vi "TPSConnect2_Test.vi"() -> ()   [LabVIEW 2009]
panel:
  in  "stop":bool
  out "Array":dbl[](array[numeric])
  in  "error in (no error)":errorcluster
  out "error out":errorcluster
  in  "ip":string
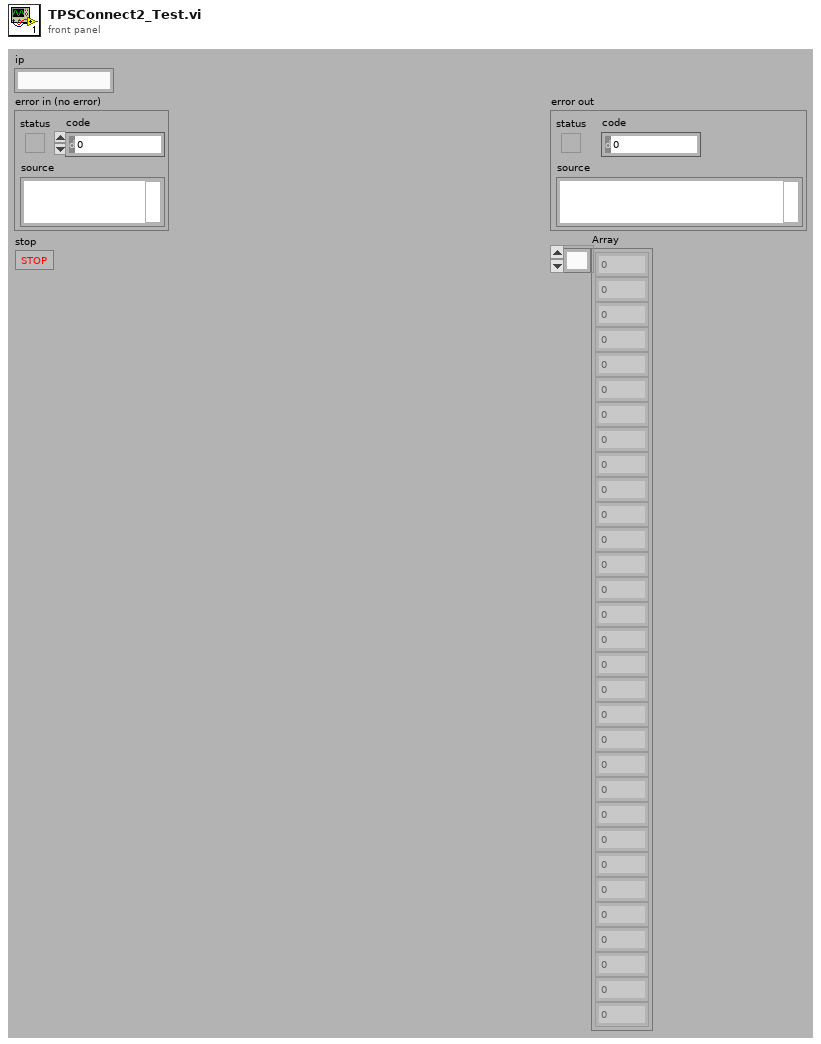
[diagram p1: front panel]
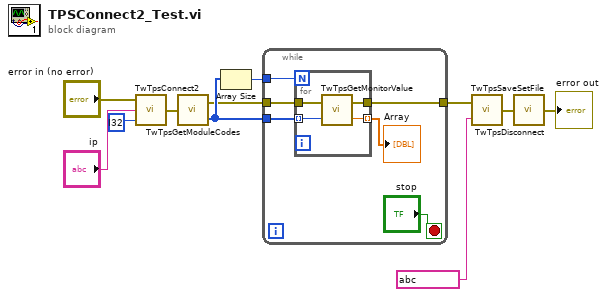
[diagram p0: block diagram]
diagram:
  n1 = call "TwTpsConnect2.vi"("type"=i32 ?, "ip"="ip", "error in (no error)"="error in (no error)") -> ("error out"=w9:errorcluster)
  n2 = call "TwTpsGetModuleCodes.vi"("error in (no error)"=w9) -> ("error out"=w5:errorcluster, "moduleCodeBuffer"=w6:i32[])
  n3 = Array Size(array=w6) -> (size(s)=w7:i32)
  n4 = while {
    tunnel: w7 -> [w17]
    tunnel: w6 -> [w16]
    tunnel: w5 -> [w15]
    tunnel: [w14] -> w3
    stop <- "stop" stop-if-true
    n5 = for {
      N: w17 -> [_]
      tunnel: w16 -> [w19] mode=indexing
      tunnel: w15 -> [w21]
      tunnel: [w20] -> w14
      tunnel: [w18] -> w12 mode=indexing
      n6 = call "TwTpsGetMonitorValue.vi"("moduleCode"=w19, "error in (no error)"=w21) -> ("value"=w18:dbl, "error out"=w20:errorcluster)
    }
    "Array" <- w12
  }
  n7 = call "TwTpsSaveSetFile.vi"("setFile"=string ?, "error in (no error)"=w3) -> ("error out"=w2:errorcluster)
  n8 = call "TwTpsDisconnect.vi"("error in (no error)"=w2) -> ("error out"=→"error out":errorcluster)
